vi "photon.vi"() -> ()   [LabVIEW 2023]
uses:
  <vilib>/Rock Robotics/WPI/ThirdParty/JAS_Junk/TrajLib/TypeDef/POSE3D.ctl
  <vilib>/Rock Robotics/WPI/ThirdParty/JAS_Junk/TrajLib/TypeDef/TRANSLATION3D.ctl
  <vilib>/Rock Robotics/WPI/ThirdParty/JAS_Junk/TrajLib/TypeDef/ROTATION3D.ctl
  <vilib>/Rock Robotics/WPI/ThirdParty/JAS_Junk/TrajLib/TypeDef/QUATERNION.ctl
  <vilib>/Rock Robotics/WPI/ThirdParty/PhotonPoseStrategy_ENUM.ctl
  <vilib>/Rock Robotics/WPI/ThirdParty/PhotonVisionLib/PhotonVisionLib.lvlib
  <vilib>/Rock Robotics/WPI/ThirdParty/JAS_Junk/TrajLib/Trajectory_Library.lvlib
panel:
  out "IsConnected":bool
  out "New Pose Found":bool
  out "EstimatedPose3d":T1={"Translation3d"={"X"=0.0, "Y"=0.0, "Z"=0.0}, "Rotation3d"={"Q_quaternion"={"R"=1.0, "V"=[0.0, 0.0, 0.0]}}} {"Translation3d"."Z" format="%14.3f"; "Translation3d"."Y" format="%14.3f"; "Translation3d"."X" format="%14.3f"}
  out "TimeStamp_Seconds":dbl
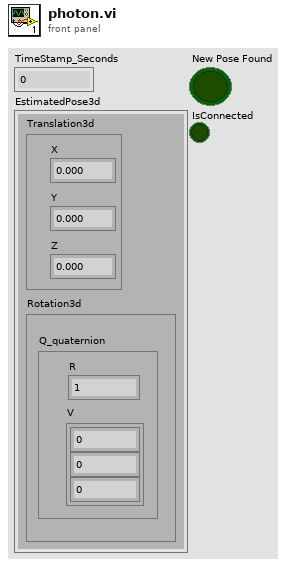
[diagram p1: front panel]
types:
  T1 = typedef "Trajectory_Library.lvlib/POSE3D.ctl" = cluster{"Translation3d":T2, "Rotation3d":T3}
  T2 = typedef "Trajectory_Library.lvlib/TRANSLATION3D.ctl" = cluster{"X":dbl, "Y":dbl, "Z":dbl}
  T3 = typedef "Trajectory_Library.lvlib/ROTATION3D.ctl" = cluster{"Q_quaternion":T4}
  T4 = typedef "Trajectory_Library.lvlib/QUATERNION.ctl" = cluster{"R":dbl, "V":dbl[]}
  T5 = enum16{"2022 Rapid React", "2023 Charged Up", "2024 Crescendo"}
  T6 = typedef "PhotonVisionLib.lvlib/PhotonPoseStrategy_ENUM.ctl" = enum16{"LOWEST_AMBIGUITY", "CLOSEST_TO_CAMERA_HEIGHT", "CLOSEST_TO_REFERENCE_POSE", "CLOSEST_TO_LAST_POSE", "AVERAGE_BEST_TARGETS", "MULTI_TAG_PNP_ON_COPROCESSOR", "MULTI_TAG_PNP_ON_RIO"}
  T7 = typedef "Trajectory_Library.lvlib/TRANSFORM3D.ctl" = cluster{"TRANSLATION3D":T2, "ROTATION3D":T3, "XF":bool}
  T8 = typedef "PhotonVisionLib.lvlib/PhotonPipelineResultType.ctl" = cluster{"TargetCount":i32, "Latency_MilliSec":dbl, "Targets":T9[], "TimeStampSec":dbl, "PhotonMultiTargetPNPResult":T11}
  T9 = typedef "PhotonVisionLib.lvlib/PhotonTrackedTargetType.ctl" = cluster{"Yaw":dbl, "Pitch":dbl, "Area":dbl, "Skew":dbl, "MinAreaRectCorners":T10[], "BestCameraToTarget":T7, "FiiducialId":i32, "AltCameraToTarget":T7, "PoseAmbiguity":dbl, "DetectedCorners":T10[]}
  T10 = typedef "PhotonVisionLib.lvlib/TargetCornerType.ctl" = cluster{"X":dbl, "Y":dbl}
  T11 = typedef "PhotonVisionLib.lvlib/PhotonMultiTargetPNPResultType.ctl" = cluster{"PhotonPNPResult":T12, "FiducialIDsUsed":i16[]}
  T12 = typedef "PhotonVisionLib.lvlib/PhotonPNPResultType.ctl" = cluster{"IsPresent":bool, "bestReprojErr":dbl, "altReprojErr":dbl, "ambiguity":dbl, "Best":T7, "Alt":T7}
  T13 = typedef "PhotonVisionLib.lvlib/PhotonPoseEstimator_Configuration.ctl" = cluster{"Primary Strategy":T6, "Camera":string, "Initial Pose":T1, "HighestAmbiguity":dbl, "Use Custom Field":bool, "Custom AprilTag Field":T14, "RobotToCamera":T7, "FallBack Strategy":T6, "BaseNTName":string, "AprilTagField":enum16{"2022 Rapid React", "2023 Charged Up", "2024 Crescendo"}}
  T14 = typedef "Trajectory_Library.lvlib/AprilTagFieldLayout.ctl" = cluster{"AprilTagMap":map{i32, T15}, "FieldLength":dbl, "FieldWidth":dbl, "OriginPosition ":T16, "OriginPose3d":T1}
  T15 = typedef "Trajectory_Library.lvlib/AprilTag.ctl" = cluster{"ID":i32, "POSE3D":T1}
  T16 = typedef "Trajectory_Library.lvlib/AprilTagFieldLayoutOrignPosition_ENUM.ctl" = enum16{"kBlueAllianceWallRightSide,", "kRedAllianceWallRightSide,"}
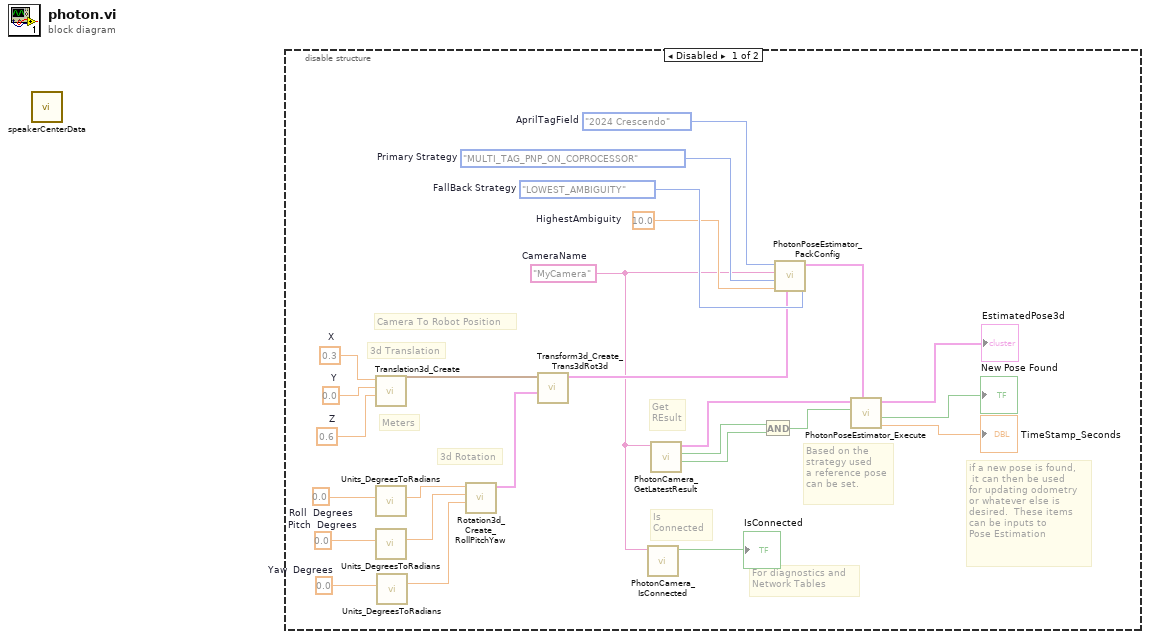
[diagram p0: block diagram]
diagram:
  n1 = call "speakerCenterData.vi"() -> ()  [unwired: 7 in, 4 out]
  n2 = disable-structure shown="Disabled" {
    frame Disabled {
      w22 = T5."2024 Crescendo"  # AprilTagField
      w21 = PhotonPoseStrategy_ENUM."LOWEST_AMBIGUITY"  # FallBack Strategy
      w13 = 0.0  # Roll  Degrees
      w12 = 0.0  # Pitch  Degrees
      w11 = 0.0  # Yaw  Degrees
      w5 = 0.6  # Z
      w6 = 0.3  # X
      w7 = 0.0  # Y
      w4 = 10.0  # HighestAmbiguity
      w3 = PhotonPoseStrategy_ENUM."MULTI_TAG_PNP_ON_COPROCESSOR"  # Primary Strategy
      w2 = "MyCamera"  # CameraName
      # "Based on the\nstrategy used\na reference pose\ncan be set."
      # "For diagnostics and \nNetwork Tables"
      # "if a new pose is found, \n it can then be used\nfor updating odometry\nor whatever else is \ndesired.  These items\ncan be inputs to\nPose Estimation"
      # "Meters"
      # "Camera To Robot Position"
      # "3d Rotation"
      # "3d Translation"
      # "Is\nConnected"
      # "Get\nREsult"
      n3 = call <vilib>:"Translation3d_Create.vi"("Z"=w5, "Y"=w7, "X"=w6) -> ("TRANSLATION3D"=w14:T2)  [unwired: 8 in]
      n4 = call <vilib>:"Units_DegreesToRadians.vi"("Degrees"=w13) -> ("Radians"=w10:dbl)  [unwired: 10 in]
      n5 = call <vilib>:"Units_DegreesToRadians.vi"("Degrees"=w12) -> ("Radians"=w9:dbl)  [unwired: 10 in]
      n6 = call <vilib>:"Units_DegreesToRadians.vi"("Degrees"=w11) -> ("Radians"=w8:dbl)  [unwired: 10 in]
      n7 = call <vilib>:"Rotation3d_Create_RollPitchYaw.vi"("Yaw"=w8, "Pitch"=w9, "Roll"=w10) -> ("Rotation3d"=w15:T3)  [unwired: 8 in]
      n8 = call <vilib>:"Transform3d_Create_Trans3dRot3d.vi"("Rotation3d"=w15, "Translation3d"=w14) -> ("Transform3d"=w16:T7)  [unwired: 9 in]
      n9 = call <vilib>:"PhotonCamera_IsConnected.vi"("CameraName"=w2) -> ("IsConnected"=→"IsConnected":bool)  [unwired: 9 in, 1 out]
      n10 = call <vilib>:"PhotonCamera_GetLatestResult.vi"("CameraName"=w2) -> ("New Data"=w20:bool, "HasTargets"=w19:bool, "PipelineResult"=w17:T8)  [unwired: 7 in, 1 out]
      n11 = And(x=w19, y=w20) -> (x .and. y?=w18:bool)
      n12 = call <vilib>:"PhotonPoseEstimator_PackConfig.vi"("FallBack Strategy"=w21, "RobotToCamera"=w16, "HighestAmbiguity"=w4, "PirmaryStrategy"=w3, "Camera"=w2, "AprilTagField"=w22) -> ("PoseEstimator_Configuration"=w1:T13)  [unwired: 5 in]
      n13 = call <vilib>:"PhotonPoseEstimator_Execute.vi"("Configuration"=w1, "PIpeline Has \nNew Results"=w18, "PipelineResult"=w17) -> ("TimeStamp_Seconds"=→"TimeStamp_Seconds":dbl, "New Pose Found"=→"New Pose Found":bool, "EstimatedPose3d"=→"EstimatedPose3d":T1)  [unwired: 2 in, 4 out]
    }
    frame Enabled {
    }
  }
